vi "State_machine.vi"() -> ()   [LabVIEW 2022 SP3]
uses:
  SM_States.ctl
  SM_Data.ctl
panel:
  out "Beer Level [ml]":dbl(slide) scale=0.0..500.0
  in  "Draught Level [ml]":dbl(slide) scale=0.0..50.0
  in  "Stop":bool
  in  "Drink":bool
  in  "SM_Data":T1={"Beer Level"=500.0}
  in  "SM_States":T2=enum."Init"
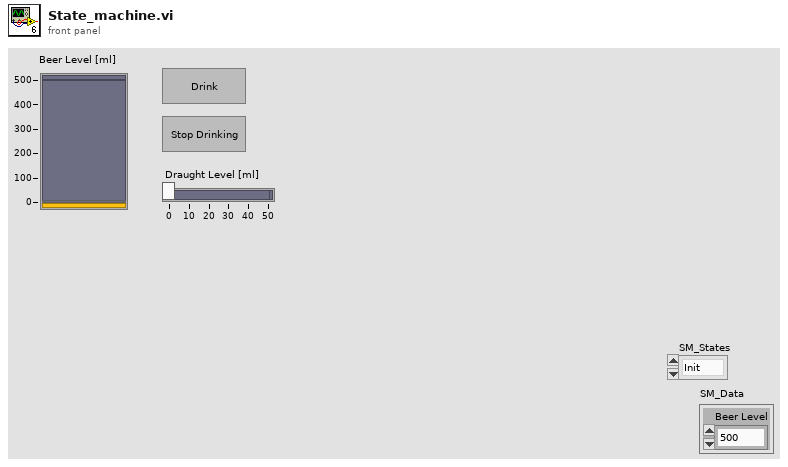
[diagram p1: front panel]
types:
  T1 = typedef "SM_Data.ctl" = cluster{"Beer Level":dbl}
  T2 = typedef "SM_States.ctl" = enum16{"Stop", "Modify Level", "Idle", "Init"}
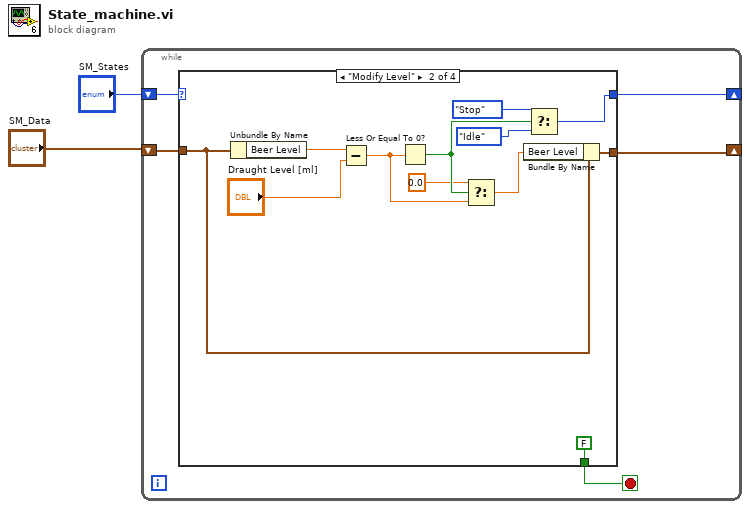
[diagram p0: block diagram]
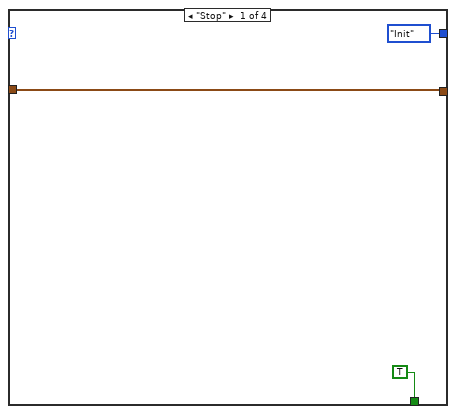
[diagram p2: hidden frame]
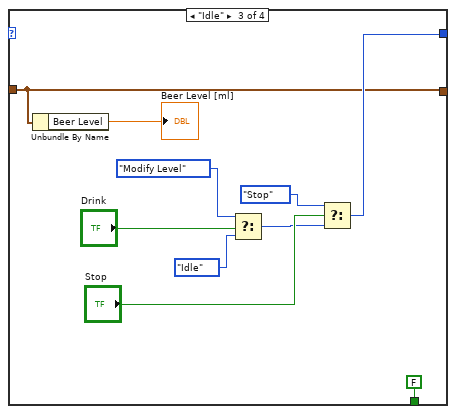
[diagram p3: hidden frame]
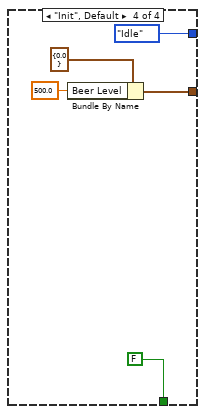
[diagram p4: hidden frame]
diagram:
  n1 = while {
    shift-right: [w6] -> _
    shift-left: "SM_States" -> [w7]
    shift-right: [w5] -> _
    shift-left: "SM_Data" -> [w3]
    stop <- w4 stop-if-true
    n2 = case shown="\"Modify Level\"" w7 {
      tunnel: [SM_States."Init" ("SM_States") w19 w26 SM_States."Idle" ("SM_States")] -> w6
      tunnel: [w8 w16 w24 w34] -> w5
      tunnel: [TRUE FALSE FALSE FALSE] -> w4
      tunnel: w3 -> [w8 w17 w24 _]
      frame "Stop" {
      }
      frame "Modify Level" {
        n3 = Unbundle By Name(w17) -> ("Beer Level"=w22:dbl)
        n4 = Subtract(x=w22, y="Draught Level [ml]") -> (x-y=w13:dbl)
        n5 = Less Or Equal To 0?(x=w13) -> (x <= 0?=w14:bool)
        n6 = Select(t=0.0, s=w14, f=w13) -> (s? t:f=w11:dbl)
        n7 = Bundle By Name(cluster=w17, "Beer Level"=w11) -> (w16:T1)
        n8 = Select(t=SM_States."Stop" ("SM_States"), s=w14, f=SM_States."Idle") -> (s? t:f=w19:T2)
      }
      frame "Idle" {
        n9 = Unbundle By Name(w24) -> ("Beer Level"=→"Beer Level [ml]":dbl)
        n10 = Select(t=SM_States."Modify Level" ("SM_States"), s="Drink", f=SM_States."Idle" ("SM_States")) -> (s? t:f=w30:T2)
        n11 = Select(t=SM_States."Stop" ("SM_States"), s="Stop", f=w30) -> (s? t:f=w26:T2)
      }
      frame "Init", Default {
        n12 = Bundle By Name(cluster=T1 {"Beer Level"=0.0} ("SM_Data"), "Beer Level"=500.0) -> (w34:T1)
      }
    }
  }
